vi "AcqDataStateMachine(SingleSample).vi"() -> ()   [LabVIEW 2013]
doc: "Læser 4 analoge differentierede datakanaler fra ADC'en og skriver dem til en TDMS-fil. Viser 2 af kanaler i grafer og 2 i søjler."
uses:
  Globals/DataAcqRecordPathGlobal.vi
  <vilib>/DAQmx/read.llb/DAQmx Read (Analog 1D DBL NChan 1Samp).vi
  Controls/Enum User Events.ctl
  Controls/Enum Globals.ctl
  Controls/Enum Variables.ctl
  <vilib>/DAQmx/configure/timing.llb/DAQmx Timing (Sample Clock).vi
panel:
  out "Pressure":dbl(slide) scale=0.0..300.0 scale format="%#.3g"
  out "Red Chart":dbl(graph)
  out "Temperature":dbl caption="Temp"
  out "Blue Chart":dbl(graph)
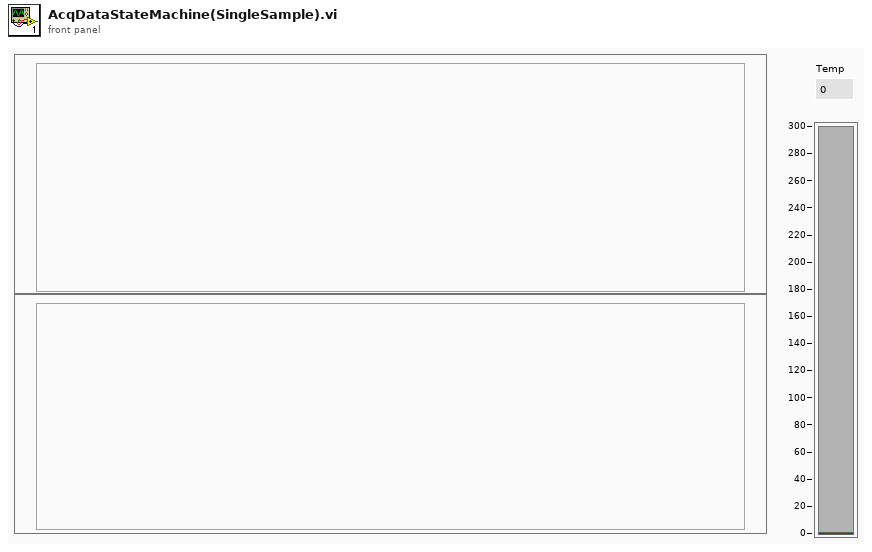
[diagram p1: front panel]
types:
  T1 = typedef "Medimatic.lvlib/Enum Globals.ctl" = enum16{"Init", "Set DataPath", "Set Freq", "Get"}
  T2 = typedef "Medimatic.lvlib/Enum Variables.ctl" = enum16{"SetAcqFilter", "GetAcqFilter", "Set Filter", "Get Filter", "Set Height", "Get Height", "Set Blue Pressure", "Get Blue Pressure", "Set Red Pressure", "Get Red Pressure", "Init", "Reset Pressure", "Set Red Cursors", "Get Red Cursors", "Set Blue Cursors", "Get Blue Cursors", "Set Language", "Get Language", "Set Active Graphs", "Get ActiveGraphs", "Set Method", "Get Method", "Set Encryption", "Get Encryption", "Set ExcelVersion", "Get ExcelVersion", "Set itemTags", "Get itemTags", "Set Attributes", "Get Attributes", "Set DICOM Avail", "Get DICOM Avail", "Set DICOM Encode", "Get DICOM Encode", "Set JournalExport", "Get JournalExport"}
  T3 = enum16{"open", "open or create", "create or replace", "create", "open (read-only)"}
  T4 = typedef "Medimatic.lvlib/Enum User Events.ctl" = enum16{"User Event", "Init"}
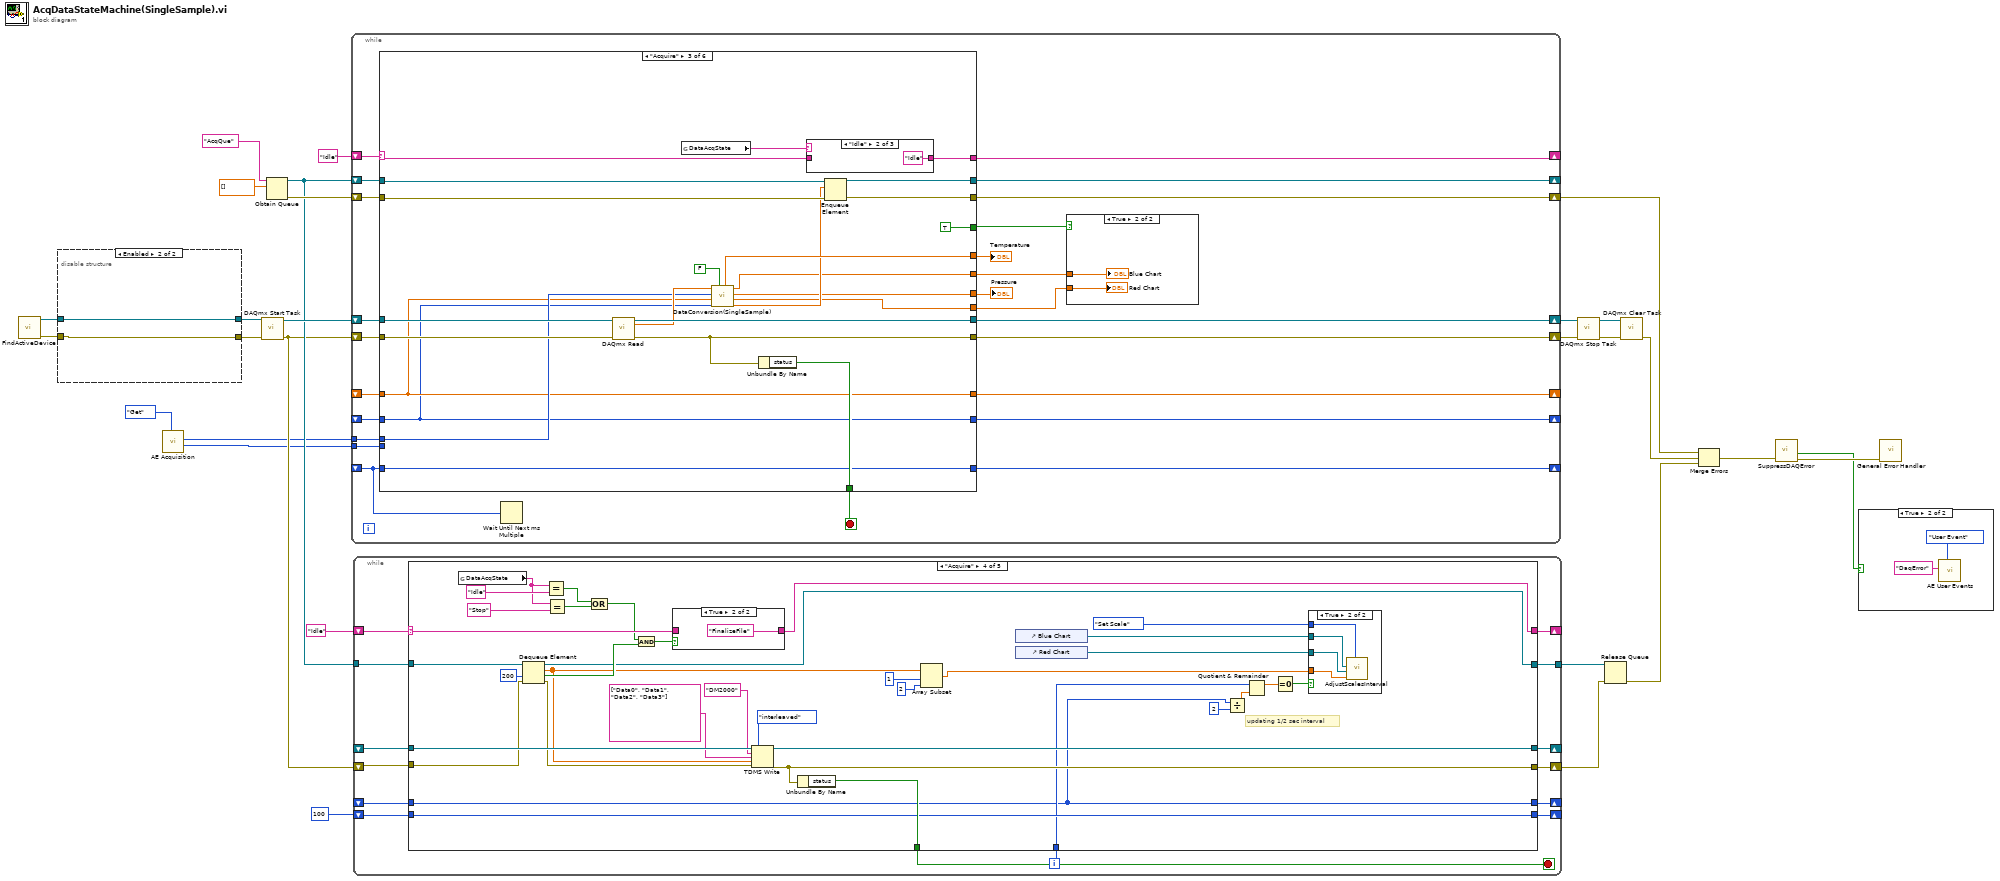
[diagram p0: block diagram]
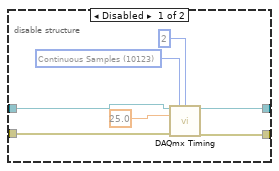
[diagram p2: hidden frame]
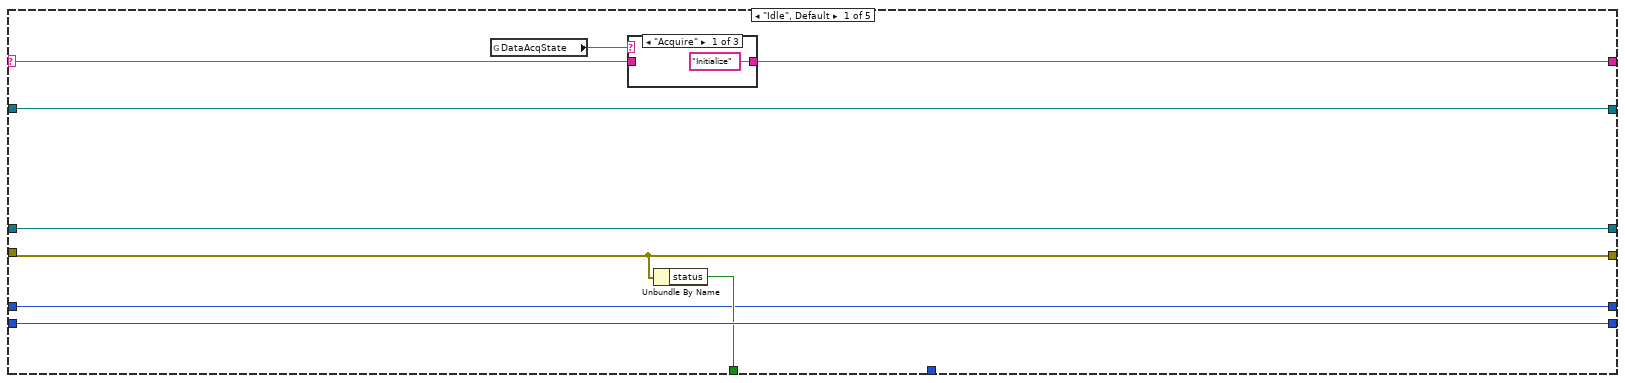
[diagram p4: hidden frame]
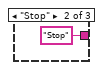
[diagram p5: hidden frame]
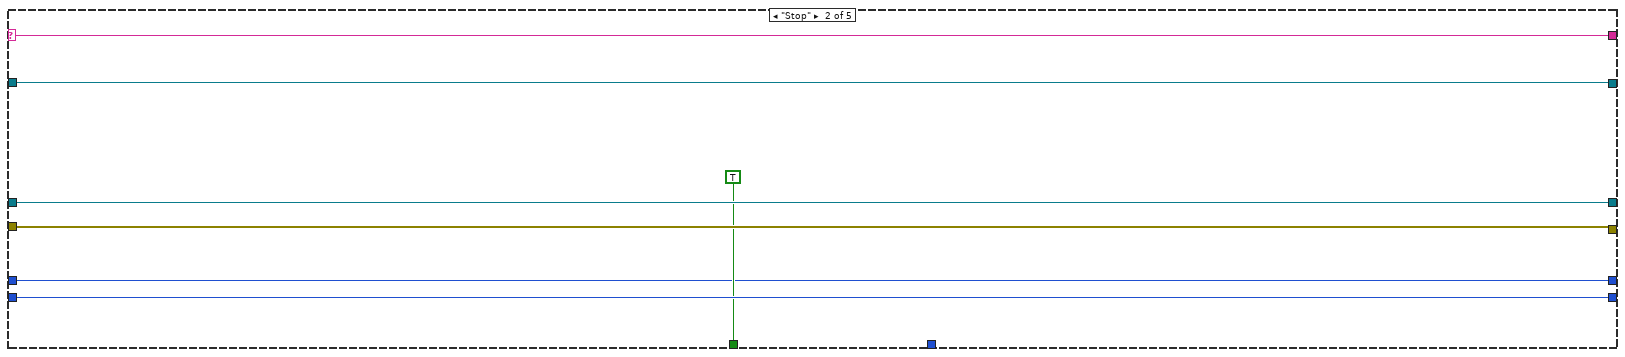
[diagram p7: hidden frame]
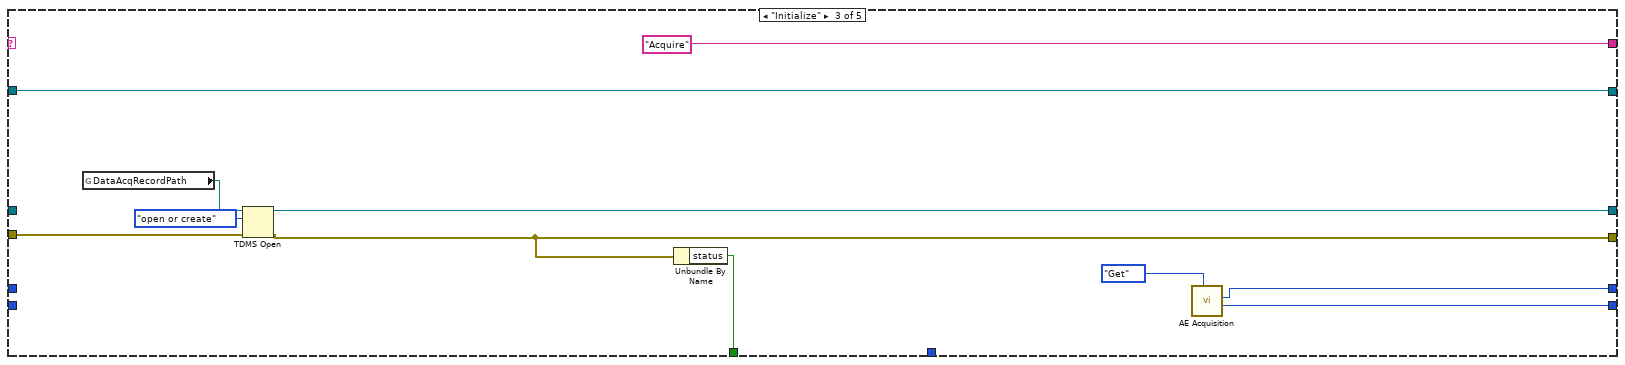
[diagram p8: hidden frame]
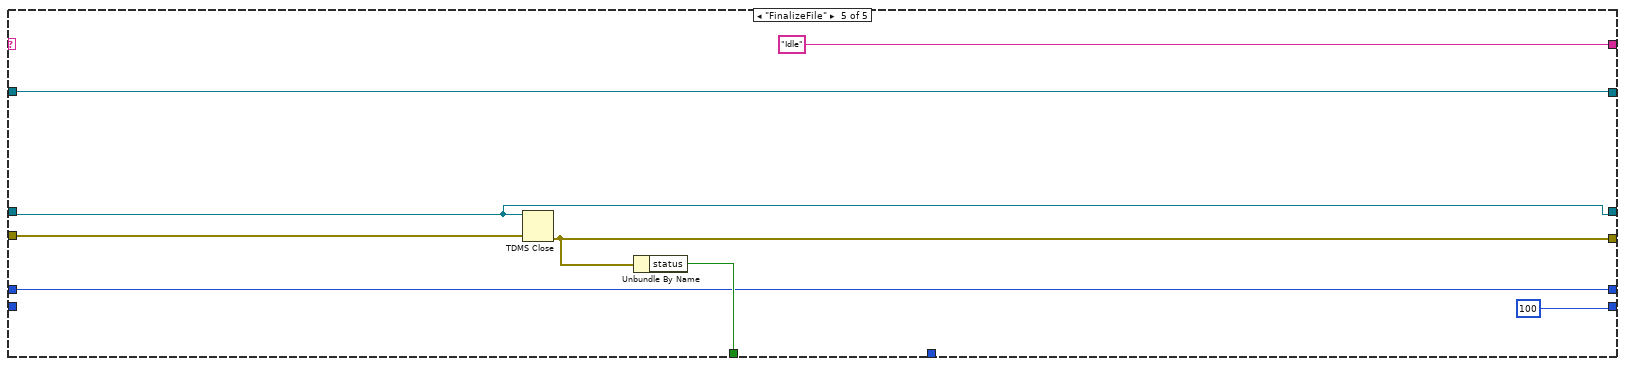
[diagram p11: hidden frame]
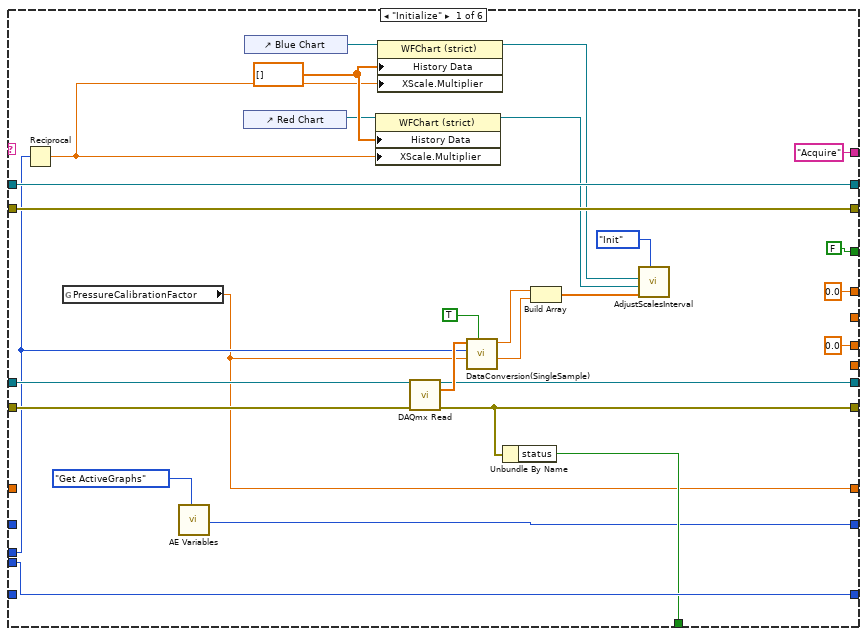
[diagram p13: hidden frame]
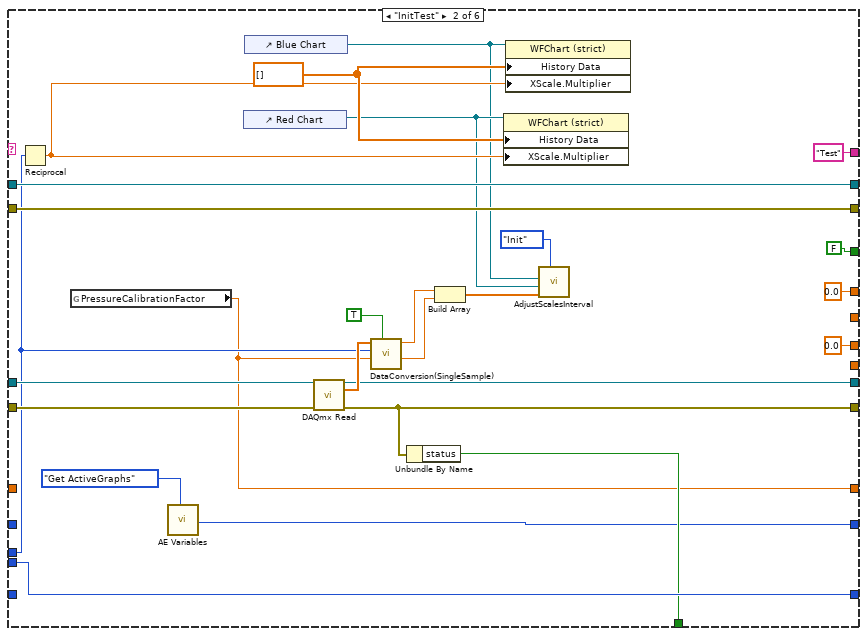
[diagram p14: hidden frame]
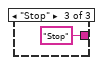
[diagram p16: hidden frame]
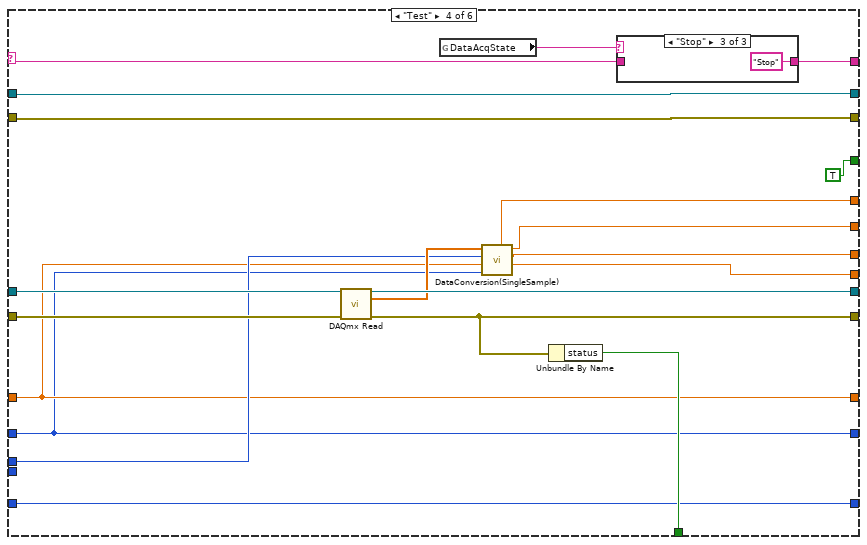
[diagram p17: hidden frame]
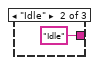
[diagram p19: hidden frame]
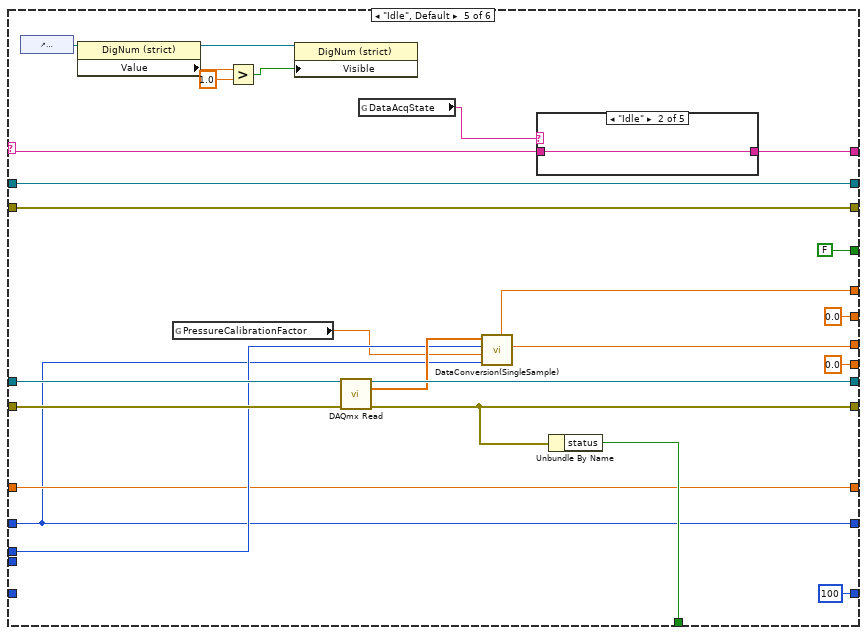
[diagram p20: hidden frame]
diagram:
  n1 = call "FindActiveDevice.vi"() -> ("error out"=w4:errorcluster, "task out"=w3:refnum<k21>)  [unwired: 10 in]
  n2 = disable-structure shown="Enabled" {
    disable-tunnel: w4 -> [w32 w36]
    disable-tunnel: w3 -> [w31 w37]
    disable-tunnel: [w30 w37] -> w2
    disable-tunnel: [w29 w36] -> w1
    frame Disabled {
      w34 = 10123 items=["Finite Samples"=10178, "Continuous Samples"=10123, "Hardware Timed Single Point"=12522] ("sample mode")
      n3 = call-poly <vilib>:"DAQmx Timing.vi"("task/channels in"=w31, "sample mode"=w34, "samples per channel"=2, "rate"=25.0, "error in"=w32) -> ("task out"=w30:refnum<k21>, "error out"=w29:errorcluster)  [unwired: 9 in]
    }
    frame Enabled {
    }
  }
  n4 = call "AE Acquisition.vi"("Action"=Enum_Globals."Get") -> ("Period(ms)"=w8:i32, "Freq Out"=w9:i32)  [unwired: 7 in, 2 out]
  n5 = call <vilib>:"DAQmx Start Task.vi"("task/channels in"=w2, "error in"=w1) -> ("task out"=w24:refnum<k21>, "error out"=w15:errorcluster)  [unwired: 12 in]
  n6 = Obtain Queue(name (unnamed)="AcqQue", element data type=dbl[] []) -> (queue out=w21:refnum<queue>, error out=w23:errorcluster)  [unwired: 3 in, 1 out]
  n7 = while {
    shift-right: [w60] -> w25
    shift-left: w24 -> [w61]
    shift-right: [w40] -> w28
    shift-left: w15 -> [w59]
    shift-right: [w48] -> _
    shift-left: _ -> [w57]
    shift-right: [w55] -> _
    shift-left: w21 -> [w56]
    shift-right: [w54] -> w11
    shift-left: w23 -> [w53]
    shift-right: [w51] -> _
    shift-left: "Idle" -> [w52]
    tunnel: w9 -> [w47]
    tunnel: w8 -> [w46]
    shift-right: [w45] -> _
    shift-left: _ -> [w44]
    shift-right: [w39] -> _
    shift-left: _ -> [w38]
    stop <- w58 stop-if-true
    n8 = case shown="\"Acquire\"" w52 {
      selector: w52 -> [_ _ w128 w155 w183 w208]
      tunnel: [w71 w97 w141 w164 w193 w204] -> w40
      tunnel: w61 -> [w74 w100 w140 w163 w192 w205]
      tunnel: [w75 w101 w139 w162 w191 w205] -> w60
      tunnel: w59 -> [w77 w103 w138 w161 w190 w204]
      tunnel: [w76 w102 w136 w159 w188 TRUE ("status")] -> w58
      tunnel: [w83 w109 w127 w147 100 w203] -> w48
      tunnel: w57 -> [_ _ w127 w147 _ w203]
      tunnel: w56 -> [w91 w117 w132 w154 w187 w207]
      tunnel: [w91 w117 w135 w154 w187 w207] -> w55
      tunnel: [w90 w116 w134 w153 w186 w206] -> w54
      tunnel: w53 -> [w90 w116 w133 w153 w186 w206]
      tunnel: [0.0 0.0 w123 w150 w180 _] -> w50
      tunnel: [0.0 ("Temperature") 0.0 ("Temperature") w131 w158 w185 _] -> w49
      tunnel: ["Acquire" "Test" w129 w156 w181 w208] -> w51
      tunnel: [_ _ w125 w151 0.0 ("Blue Data") _] -> w41
      tunnel: [_ _ w124 w152 0.0 ("Red Data") _] -> w42
      tunnel: [FALSE FALSE TRUE TRUE FALSE FALSE] -> w43
      tunnel: w47 -> [w69 w95 w121 w148 w171 _]
      tunnel: w46 -> [w83 w109 _ _ _ _]
      tunnel: [w68 w94 w120 w146 w170 w200] -> w45
      tunnel: w44 -> [_ _ w120 w146 w170 w200]
      tunnel: [w64 w92 w119 w145 w168 w199] -> w39
      tunnel: w38 -> [_ _ w119 w145 w168 w199]
      frame "Initialize" {
        w85 = dbl[] [] ("Value")
        n9 = Reciprocal(x=w69) -> (1/x=w84:dbl)
        n10 = global read "DataAcqRecordPathGlobal.vi" "PressureCalibrationFactor"() -> (w68:dbl)
        n11 = call "AE Variables.vi"("Action"=Enum_Variables."Get ActiveGraphs") -> ("RingOut"=w64:u16)  [unwired: 11 in, 7 out]
        n12 = control-ref of="Red Chart"() -> (w73:refnum<vi>)
        n13 = control-ref of="Blue Chart"() -> (w72:refnum<vi>)
        n14 = property class="WFChart (strict)"(reference=w73, "History Data"=w85, "XScale.Multiplier"=w84) -> (reference out=w67:refnum<vi>)  [unwired: 1 in, 1 out]
        n15 = property class="WFChart (strict)"(reference=w72, "History Data"=w85, "XScale.Multiplier"=w84) -> (reference out=w66:refnum<vi>)  [unwired: 1 in, 1 out]
        n16 = call-poly <vilib>:"DAQmx Read.vi"("task/channels in"=w74, "error in"=w77) -> ("task out"=w75:refnum<k21>, "data"=w82:dbl[], "error out"=w71:errorcluster)  [unwired: 11 in]
        n17 = call "DataConversion(SingleSample).vi"(1:w68, 2:w69, "input cluster"=w82, "Init"=TRUE) -> ("Red Data"=w79:dbl, "Blue Data"=w80:dbl)  [unwired: 2 in, 3 out]
        n18 = Unbundle By Name(w71) -> ("status"=w76:bool)
        n19 = Build Array(w80, w79) -> (w78:dbl[])
        n20 = call "AdjustScalesInterval.vi"("Action"=enum16{"Init", "Set Scale"}."Init", "Data"=w78, "WFChart Refnum 2"=w67, "WFChart Refnum"=w66) -> ()  [unwired: 8 in]
      }
      frame "InitTest" {
        w111 = dbl[] [] ("Value")
        n21 = Reciprocal(x=w95) -> (1/x=w110:dbl)
        n22 = global read "DataAcqRecordPathGlobal.vi" "PressureCalibrationFactor"() -> (w94:dbl)
        n23 = call "AE Variables.vi"("Action"=Enum_Variables."Get ActiveGraphs") -> ("RingOut"=w92:u16)  [unwired: 11 in, 7 out]
        n24 = control-ref of="Red Chart"() -> (w99:refnum<vi>)
        n25 = control-ref of="Blue Chart"() -> (w98:refnum<vi>)
        n26 = call-poly <vilib>:"DAQmx Read.vi"("task/channels in"=w100, "error in"=w103) -> ("task out"=w101:refnum<k21>, "data"=w108:dbl[], "error out"=w97:errorcluster)  [unwired: 11 in]
        n27 = call "DataConversion(SingleSample).vi"(1:w94, 2:w95, "input cluster"=w108, "Init"=TRUE) -> ("Red Data"=w105:dbl, "Blue Data"=w106:dbl)  [unwired: 2 in, 3 out]
        n28 = Unbundle By Name(w97) -> ("status"=w102:bool)
        n29 = Build Array(w106, w105) -> (w104:dbl[])
        n30 = property class="WFChart (strict)"(reference=w99, "History Data"=w111, "XScale.Multiplier"=w110) -> ()  [unwired: 1 in, 2 out]
        n31 = property class="WFChart (strict)"(reference=w98, "History Data"=w111, "XScale.Multiplier"=w110) -> ()  [unwired: 1 in, 2 out]
        n32 = call "AdjustScalesInterval.vi"("Action"=enum16{"Init", "Set Scale"}."Init", "Data"=w104, "WFChart Refnum 2"=w99, "WFChart Refnum"=w98) -> ()  [unwired: 8 in]
      }
      frame "Acquire" {
        n33 = call-poly <vilib>:"DAQmx Read.vi"("task/channels in"=w140, "error in"=w138) -> ("task out"=w139:refnum<k21>, "data"=w137:dbl[], "error out"=w141:errorcluster)  [unwired: 11 in]
        n34 = global read "DataAcqRecordPathGlobal.vi" "DataAcqState"() -> (w130:string)
        n35 = call "DataConversion(SingleSample).vi"(0:w119, 1:w120, 2:w121, "input cluster"=w137, "Init"=FALSE) -> ("Temperature"=w131:dbl, "All Data"=w126:dbl[], "Red Data"=w124:dbl, "Pressure"=w123:dbl, "Blue Data"=w125:dbl)  [unwired: 1 in]
        n36 = Unbundle By Name(w141) -> ("status"=w136:bool)
        n37 = case shown="\"Idle\"" w130 {
          tunnel: [w142 "Idle" "Stop"] -> w129
          tunnel: w128 -> [w142 _ _]
          frame "False", Default {
          }
          frame "Idle" {
          }
          frame "Stop" {
          }
        }
        n38 = Enqueue Element(queue=w132, element=w126, error in (no error)=w133) -> (queue out=w135:refnum<queue>, error out=w134:errorcluster)  [unwired: 1 in, 1 out]
      }
      frame "Test" {
        n39 = call-poly <vilib>:"DAQmx Read.vi"("task/channels in"=w163, "error in"=w161) -> ("task out"=w162:refnum<k21>, "data"=w160:dbl[], "error out"=w164:errorcluster)  [unwired: 11 in]
        n40 = global read "DataAcqRecordPathGlobal.vi" "DataAcqState"() -> (w157:string)
        n41 = call "DataConversion(SingleSample).vi"(0:w145, 1:w146, 2:w148, "input cluster"=w160) -> ("Temperature"=w158:dbl, "Red Data"=w152:dbl, "Pressure"=w150:dbl, "Blue Data"=w151:dbl)  [unwired: 2 in, 1 out]
        n42 = Unbundle By Name(w164) -> ("status"=w159:bool)
        n43 = case shown="\"Stop\"" w157 {
          tunnel: [w165 "Idle" "Stop"] -> w156
          tunnel: w155 -> [w165 _ _]
          frame "False", Default {
          }
          frame "Idle" {
          }
          frame "Stop" {
          }
        }
      }
      frame "Idle", Default {
        n44 = control-ref of="Temperature"() -> (w176:refnum<vi>)
        n45 = property class="DigNum (strict)"(reference=w176) -> (reference out=w175:refnum<vi>, "Value"=w174:dbl)  [unwired: 1 in, 1 out]
        n46 = global read "DataAcqRecordPathGlobal.vi" "PressureCalibrationFactor"() -> (w169:dbl)
        n47 = Greater?(x=w174, y=1.0) -> (0:w172:bool)
        n48 = property class="DigNum (strict)"(reference=w175, "Visible"=w172) -> ()  [unwired: 1 in, 2 out]
        n49 = call-poly <vilib>:"DAQmx Read.vi"("task/channels in"=w192, "error in"=w190) -> ("task out"=w191:refnum<k21>, "data"=w189:dbl[], "error out"=w193:errorcluster)  [unwired: 11 in]
        n50 = global read "DataAcqRecordPathGlobal.vi" "DataAcqState"() -> (w182:string)
        n51 = call "DataConversion(SingleSample).vi"(0:w168, 1:w169, 2:w171, "input cluster"=w189) -> ("Temperature"=w185:dbl, "Pressure"=w180:dbl)  [unwired: 2 in, 3 out]
        n52 = case shown="\"Idle\"" w182 {
          tunnel: w183 -> [w194 w195 _ _ _]
          tunnel: [w194 w195 "Initialize" "Stop" "InitTest"] -> w181
          frame "False", Default {
          }
          frame "Idle" {
          }
          frame "Acquire" {
          }
          frame "Stop" {
          }
          frame "Test" {
          }
        }
        n53 = Unbundle By Name(w193) -> ("status"=w188:bool)
      }
      frame "Stop" {
      }
    }
    "Pressure" <- w50
    "Temperature" <- w49
    n54 = Wait Until Next ms Multiple(millisecond multiple=w57) -> ()  [unwired: 1 out]
    n55 = case shown="True" w43 {
      tunnel: w42 -> [_ w63]
      tunnel: w41 -> [_ w62]
      frame False {
      }
      frame True {
        "Blue Chart" <- w62
        "Red Chart" <- w63
      }
    }
  }
  n56 = while {
    tunnel: w21 -> [w222]
    shift-right: [w220] -> _
    shift-left: _ -> [w221]
    shift-right: [w219] -> w13
    shift-left: w15 -> [w218]
    shift-right: [w215] -> _
    shift-left: "Idle" -> [w216]
    shift-right: [w214] -> _
    shift-left: 100 -> [w213]
    tunnel: [w212] -> w14
    shift-right: [w210] -> _
    shift-left: _ -> [w209]
    i -> [w211]
    stop <- w217 stop-if-true
    n57 = case shown="\"Acquire\"" w216 {
      selector: w216 -> [w228 w241 _ w282 _]
      tunnel: w222 -> [w226 w236 w245 w284 w298]
      tunnel: w221 -> [w230 w240 _ w287 w297]
      tunnel: [w230 w240 w247 w288 w297] -> w220
      tunnel: [w225 w239 w248 w286 w299] -> w219
      tunnel: w218 -> [w225 w239 w250 w278 w302]
      tunnel: [w224 TRUE ("status") w249 w285 w300] -> w217
      tunnel: [w229 w241 "Acquire" w267 "Idle"] -> w215
      tunnel: w213 -> [w231 w238 _ w283 _]
      tunnel: [w231 w238 w242 w283 100] -> w214
      tunnel: [w226 w236 w245 w266 w298] -> w212
      tunnel: w211 -> [_ _ _ w258 _]
      tunnel: [w223 w235 w243 w253 w295] -> w210
      tunnel: w209 -> [w223 w235 _ w253 w295]
      frame "Idle", Default {
        n58 = global read "DataAcqRecordPathGlobal.vi" "DataAcqState"() -> (w227:string)
        n59 = case shown="\"Acquire\"" w227 {
          tunnel: ["Initialize" "Stop" w234] -> w229
          tunnel: w228 -> [_ _ w234]
          frame "Acquire" {
          }
          frame "Stop" {
          }
          frame "Idle", Default {
          }
        }
        n60 = Unbundle By Name(w225) -> ("status"=w224:bool)
      }
      frame "Stop" {
      }
      frame "Initialize" {
        n61 = global read "DataAcqRecordPathGlobal.vi" "DataAcqRecordPath"() -> (w252:path)
        n62 = TDMS Open(8:w250, 10:T3."open or create" ("operation (0:open)"), 11:w252) -> (0:w248:errorcluster, 3:w247:refnum<k34>)  [unwired: 4 in]
        n63 = Unbundle By Name(w248) -> ("status"=w249:bool)
        n64 = call "AE Acquisition.vi"("Action"=Enum_Globals."Get") -> ("Period(ms)"=w242:i32, "Freq Out"=w243:i32)  [unwired: 7 in, 2 out]
      }
      frame "Acquire" {
        # "updating 1/2 sec interval"
        n65 = global read "DataAcqRecordPathGlobal.vi" "DataAcqState"() -> (w271:string)
        n66 = Dequeue Element(queue=w284, timeout in ms (-1)=200, error in (no error)=w278) -> (queue out=w266:refnum<queue>, element=w257:dbl[], timed out?=w275:bool, error out=w277:errorcluster)
        n67 = Equal?(x=w271, y="Idle") -> (x = y?=w273:bool)
        n68 = Equal?(x=w271, y="Stop") -> (x = y?=w270:bool)
        n69 = Compound Arithmetic op=OR(w273, w270) -> (w269:bool)
        n70 = And(x=w269, y=w275) -> (x .and. y?=w274:bool)
        n71 = case shown="True" w274 {
          tunnel: [w293 "FinalizeFile"] -> w267
          tunnel: w282 -> [w293 _]
          frame False {
          }
          frame True {
          }
        }
        n72 = TDMS Write(0:w287, 1:enum16{"decimated", "interleaved"}."interleaved" ("data layout (0:decimated)"), 5:"DM2000", 7:string[] ["Data0", "Data1", "Data2", "Data3"], 9:w257, 11:w277) -> (4:w288:refnum<k34>, 15:w286:errorcluster)  [unwired: 2 out]
        n73 = Unbundle By Name(w286) -> ("status"=w285:bool)
        n74 = Array Subset(array=w257, index=1, length=2) -> (w254:dbl[])
        n75 = control-ref of="Blue Chart"() -> (w265:refnum<vi>)
        n76 = control-ref of="Red Chart"() -> (w264:refnum<vi>)
        n77 = Divide(x=w253, y=2) -> (x/y=w261:dbl)
        n78 = Quotient & Remainder(x=w258, y=w261) -> (x-y*floor(x/y)=w260:dbl)  [unwired: 1 out]
        n79 = Equal To 0?(x=w260) -> (x = 0?=w259:bool)
        n80 = case shown="True" w259 {
          tunnel: w265 -> [_ w292]
          tunnel: w264 -> [_ w291]
          tunnel: w254 -> [_ w290]
          tunnel: enum16{"Init", "Set Scale"}."Set Scale" ("Action") -> [_ w289]
          frame False {
          }
          frame True {
            n81 = call "AdjustScalesInterval.vi"("Action"=w289, "Data"=w290, "WFChart Refnum 2"=w291, "WFChart Refnum"=w292) -> ()  [unwired: 8 in]
          }
        }
      }
      frame "FinalizeFile" {
        n82 = TDMS Close(8:w302, 11:w297) -> (0:w299:errorcluster)  [unwired: 1 out]
        n83 = Unbundle By Name(w299) -> ("status"=w300:bool)
      }
    }
  }
  n84 = call <vilib>:"DAQmx Stop Task.vi"("task/channels in"=w25, "error in"=w28) -> ("task out"=w27:refnum<k21>, "error out"=w26:errorcluster)  [unwired: 12 in]
  n85 = Release Queue(queue=w14, error in (no error)=w13) -> (error out=w12:errorcluster)  [unwired: 1 in, 2 out]
  n86 = call <vilib>:"DAQmx Clear Task.vi"("task in"=w27, "error in"=w26) -> ("error out"=w16:errorcluster)  [unwired: 13 in]
  n87 = Merge Errors(w11, w16, w12) -> (w7:errorcluster)
  n88 = call "SuppressDAQError.vi"("error IO"=w7) -> ("Error Out"=w6:errorcluster, "Error Filtered?"=w5:bool)  [unwired: 7 in]
  n89 = case shown="True" w5 {
    frame False {
    }
    frame True {
      n90 = call "AE User Events.vi"("Action"=Enum_User_Events."User Event", "User Event"="DaqError") -> ()  [unwired: 8 in, 2 out]
    }
  }
  n91 = call <vilib>:"General Error Handler.vi"("error in (no error)"=w6) -> ()  [unwired: 10 in, 5 out]
